vi "main.vi"() -> ()   [LabVIEW 2015]
uses:
  USB Template (LV 8.6)/Car Wash/Controls/Car Wash Indicators.ctl
  USB Template (LV 8.6)/Car Wash/Controls/Wash Options.ctl
  controls/state.ctl
  controls/wash indicators.ctl
  controls/times.ctl
  controls/timer state.ctl
panel:
  out "error out":errorcluster
  in  "error in":errorcluster
  in  "Wash Options":T1
  in  "Start":bool
  out "Elapsed Time":dbl format="%0.2f"
  in  "stop":bool
  out "Wash Entry":bool
  in  "Car Position Slider":u8(slide) max=3 scale=0.0..4.0
  out "Car Wash Indicators":T2
  # "Entry Console"
  # "Car Wash Display"
  # "Car Position Simulation"
  # "Pre-Soak\nH-P Wash\nL-P Wax\nSpot Free Rinse"
  # "Underbody Wash\nBug Remover"
  # "Tire Shine\nAir Dry"
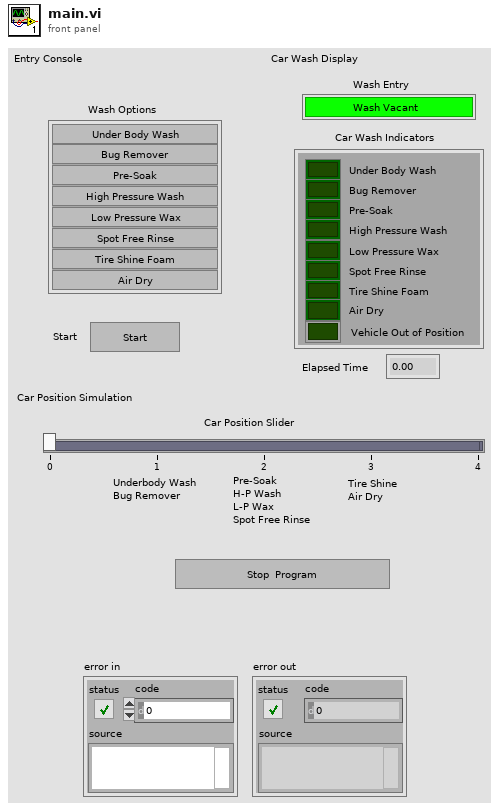
[diagram p1: front panel]
types:
  T1 = typedef "Wash Options.ctl" = cluster{"Underbody Wash":bool, "Bug Remover":bool, "Pre-Soak":bool, "High Pressure Wash":bool, "Low Pressure Wax":bool, "Spot Free Rinse":bool, "Tire Shine Foam":bool, "Air Dry":bool}
  T2 = typedef "Car Wash Indicators.ctl" = cluster{"Under Body Wash":bool, "Bug Remover":bool, "Pre-Soak":bool, "High Pressure Wash":bool, "Low Pressure Wax":bool, "Spot Free Rinse":bool, "Tire Shine Foam":bool, "Air Dry":bool, "Vehicle Out of Position":bool}
  T3 = typedef "state.ctl" = enum16{"Error", "Reset", "Exit", "Next state", "End", "Idle", "UBW", "Bug Remover", "Pre-Soak", "HPW", "LPW", "SFR", "TSF", "Air Dry", "Initialize"}
  T4 = enum8{"Enabled", "Disabled", "Disabled and Grayed Out"}
  T5 = typedef "timer state.ctl" = enum16{"Stop", "Pause", "Start"}
  T6 = typedef "wash indicators.ctl" = cluster{"Car Wash Indicators ":T2, "Wash Entry ":bool, "Elapsed Time ":dbl, "times":T7}
  T7 = typedef "times.ctl" = cluster{"Under Body Wash":dbl, "Bug Remover":dbl, "Pre-Soak":dbl, "High Pressure Wash ":dbl, "Low Pressure Wax":dbl, "Spot Free Rinse":dbl, "Tire Shine Foam":dbl, "Air Dry":dbl}
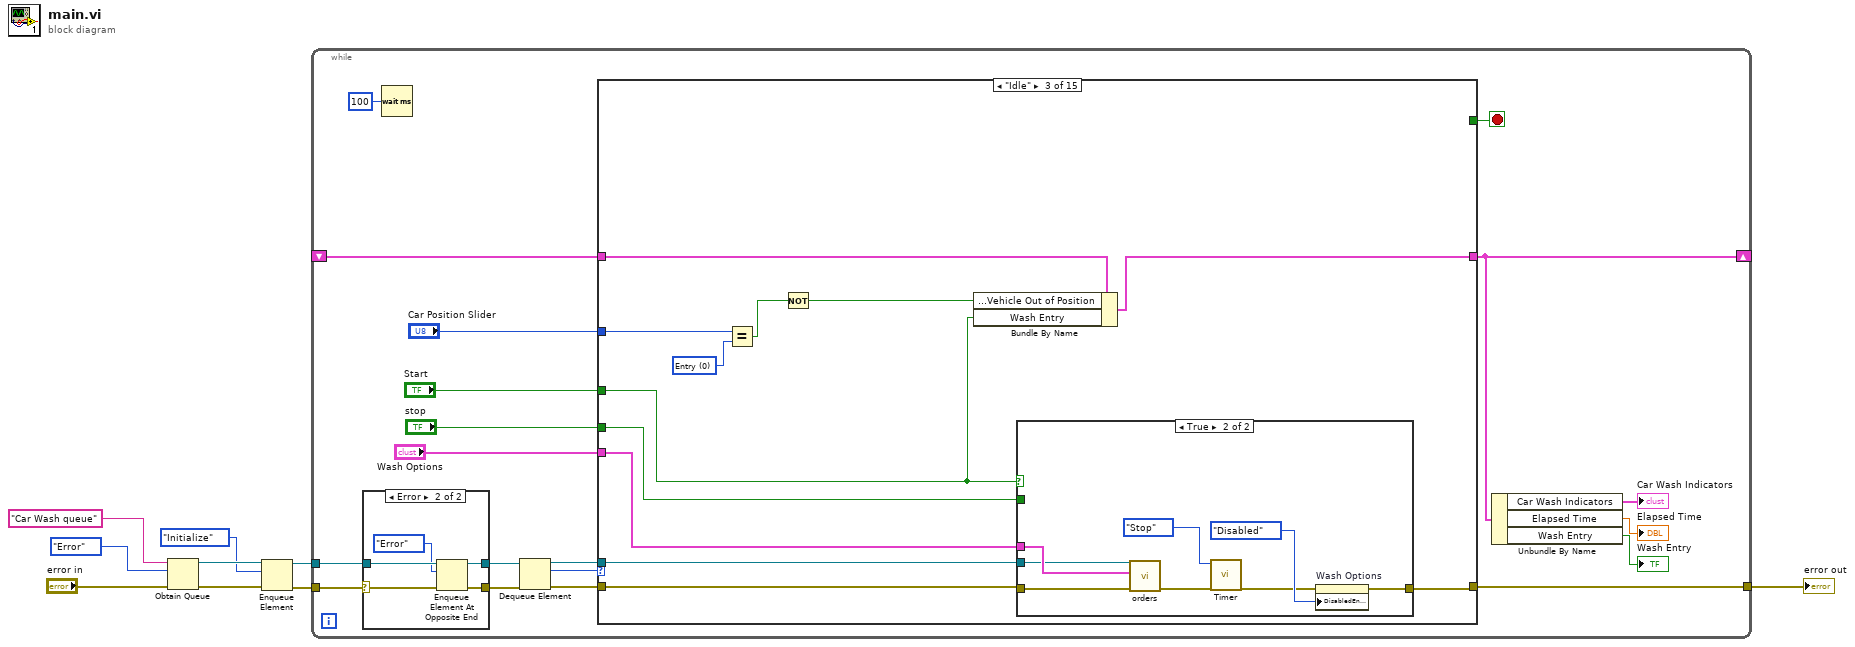
[diagram p0: block diagram]
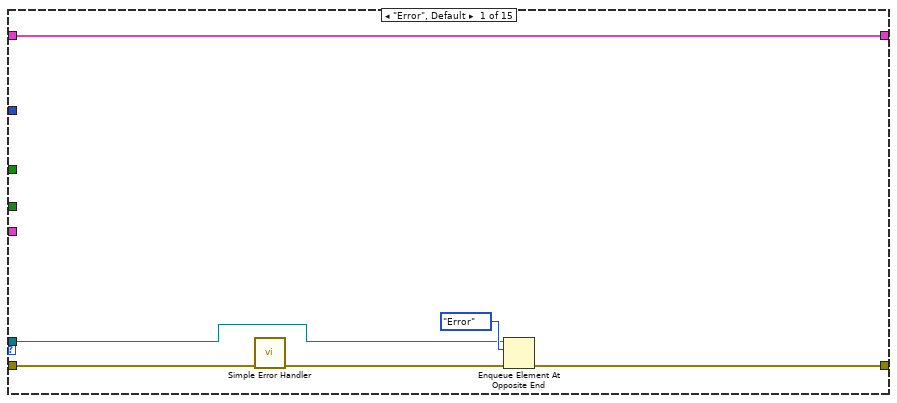
[diagram p3: hidden frame]
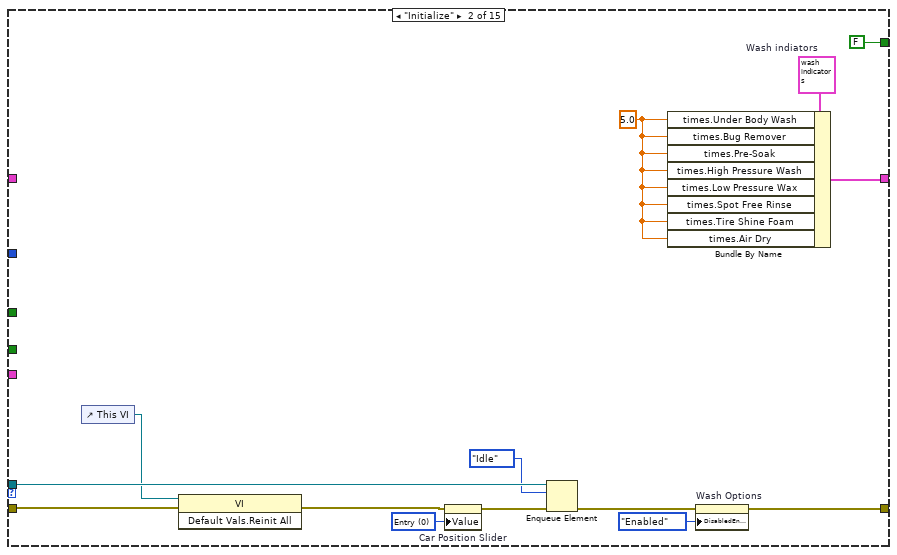
[diagram p4: hidden frame]
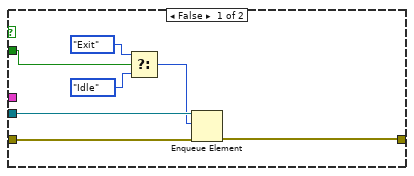
[diagram p5: hidden frame]
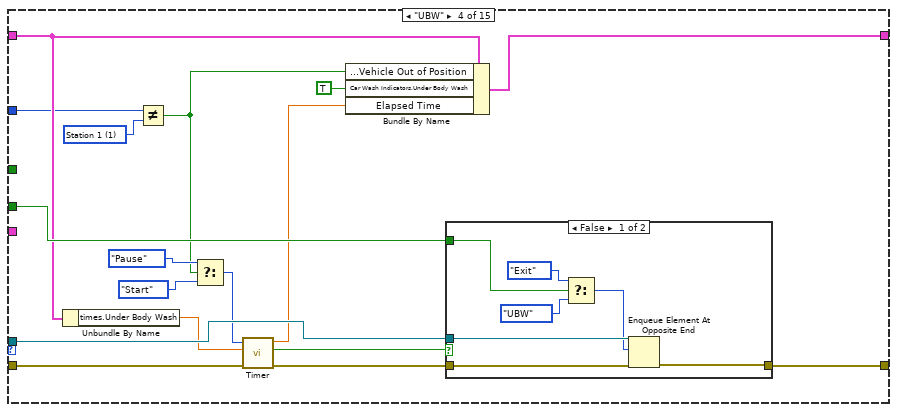
[diagram p6: hidden frame]
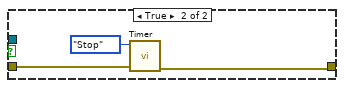
[diagram p7: hidden frame]
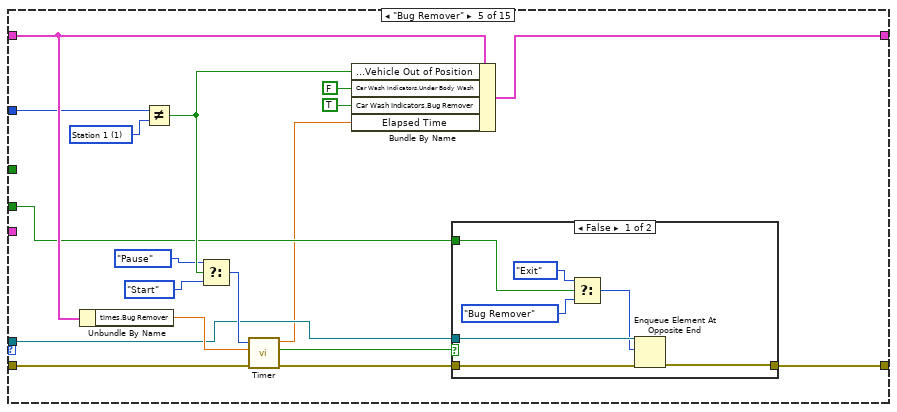
[diagram p8: hidden frame]
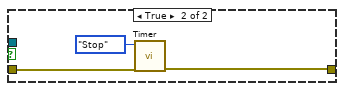
[diagram p9: hidden frame]
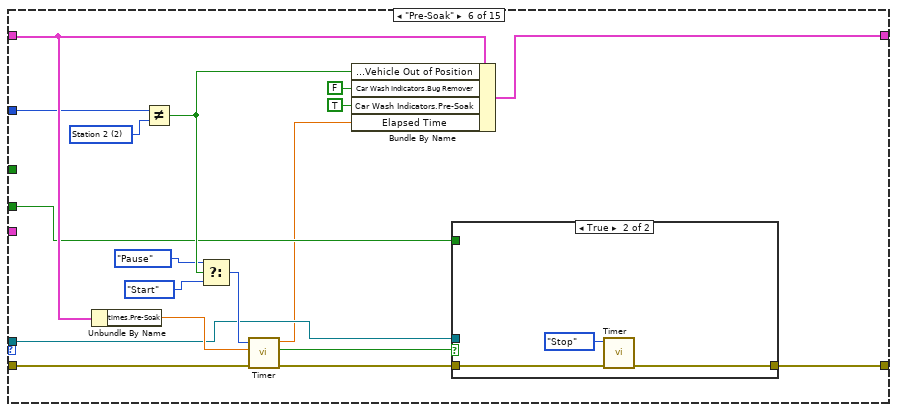
[diagram p10: hidden frame]
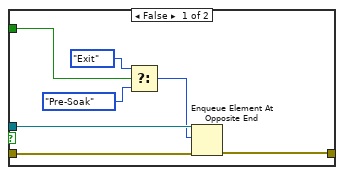
[diagram p11: hidden frame]
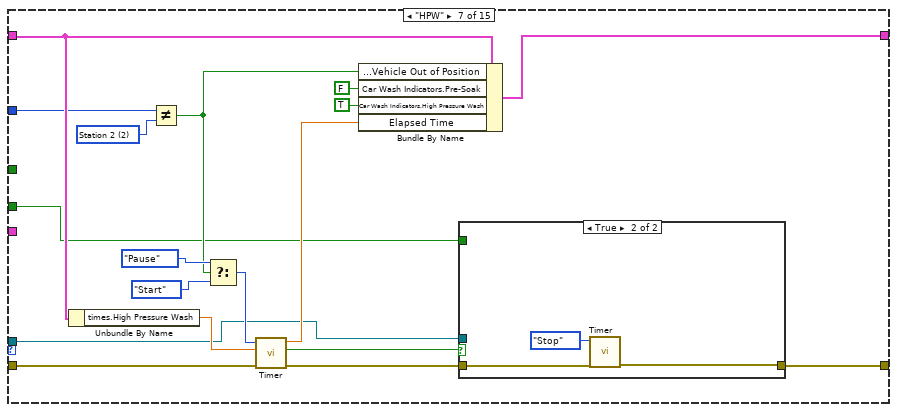
[diagram p12: hidden frame]
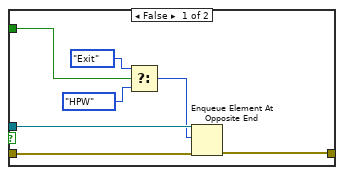
[diagram p13: hidden frame]
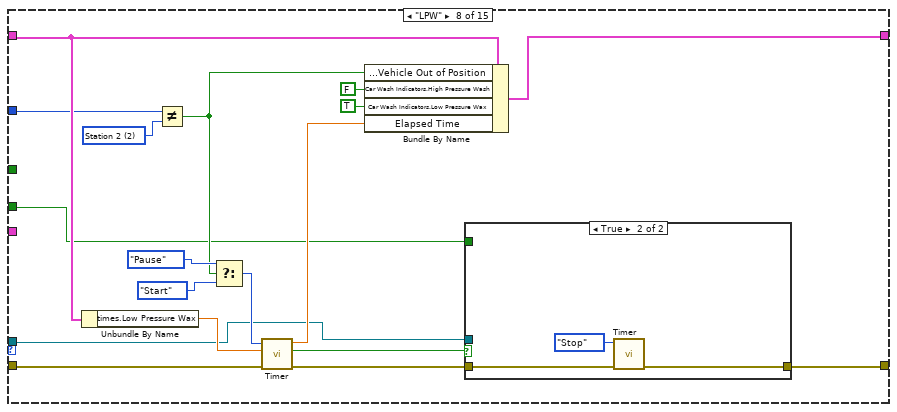
[diagram p14: hidden frame]
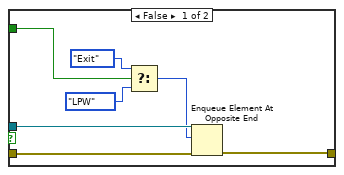
[diagram p15: hidden frame]
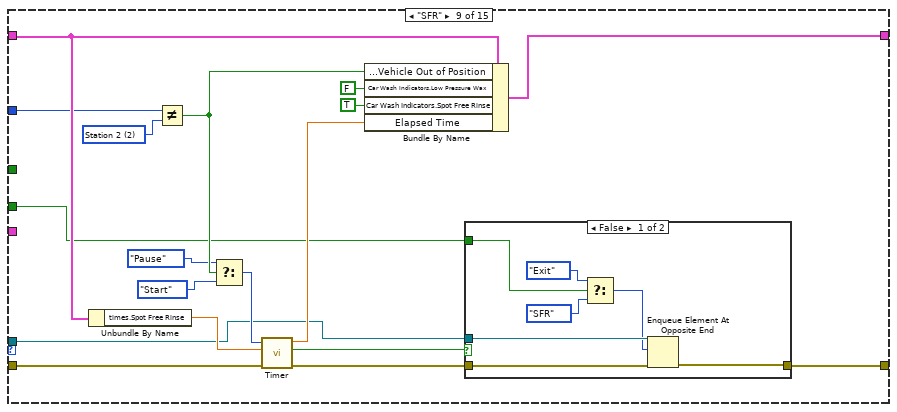
[diagram p16: hidden frame]
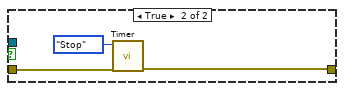
[diagram p17: hidden frame]
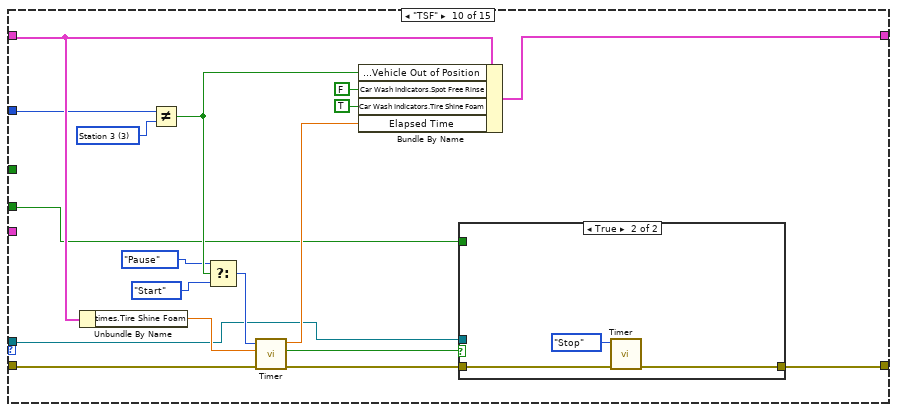
[diagram p18: hidden frame]
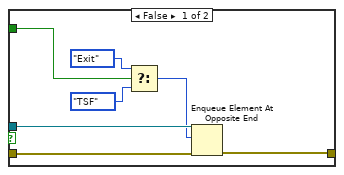
[diagram p19: hidden frame]
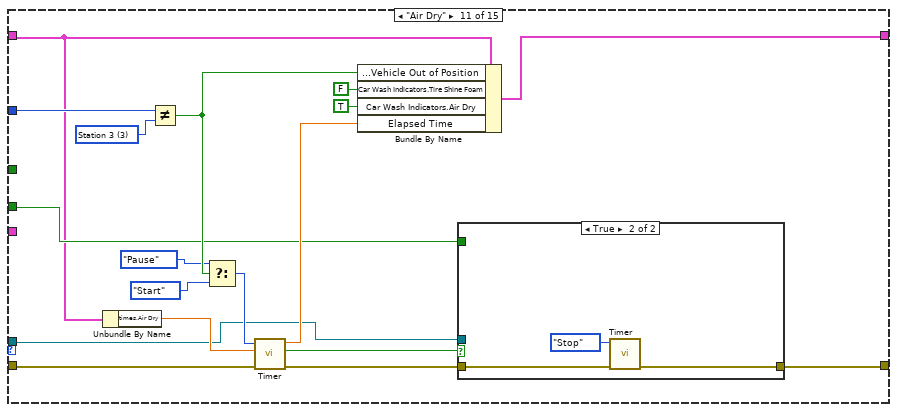
[diagram p20: hidden frame]
diagram:
  n1 = Obtain Queue(name (unnamed)="Car Wash queue", element data type=state."Error" ("state"), error in (no error)="error in") -> (queue out=w3:refnum<queue>, error out=w7:errorcluster)  [unwired: 2 in, 1 out]
  n2 = Enqueue Element(queue=w3, element=state."Initialize" ("state"), error in (no error)=w7) -> (queue out=w1:refnum<queue>, error out=w6:errorcluster)  [unwired: 1 in, 1 out]
  n3 = while {
    tunnel: [w28] -> w9
    tunnel: w6 -> [w18]
    tunnel: w1 -> [w15]
    shift-right: [w14] -> _
    shift-left: _ -> [w21]
    stop <- w24 stop-if-true
    n4 = case shown="Error" w18 {
      selector: w18 -> [w30 w35]
      tunnel: [w30 w34] -> w17
      tunnel: [w29 w33] -> w16
      tunnel: w15 -> [w29 w32]
      frame No Error {
      }
      frame Error {
        n5 = Enqueue Element At Opposite End(queue=w32, element=state."Error" ("state"), error in (no error)=w35) -> (queue out=w33:refnum<queue>, error out=w34:errorcluster)  [unwired: 1 in, 1 out]
      }
    }
    n6 = Wait (ms)(milliseconds to wait=u32 100) -> ()  [unwired: 1 out]
    n7 = Dequeue Element(queue=w16, error in (no error)=w17) -> (queue out=w26:refnum<queue>, element=w25:T3, error out=w27:errorcluster)  [unwired: 1 in, 1 out]
    n8 = case shown="\"Idle\"" w25 {
      tunnel: w27 -> [w41 w44 w66 w97 w117 w143 w171 w198 w227 w255 w284 w308 w313 w319 w347]
      tunnel: [w37 w49 w67 w99 w118 w144 w166 w196 w225 w253 w283 w308 w313 w318 w342] -> w28
      tunnel: w26 -> [w38 w52 w64 w95 w116 w142 w170 w197 w226 w254 w278 _ _ w315 w345]
      tunnel: [_ FALSE _ _ _ _ _ _ _ _ _ TRUE _ _ _] -> w24
      tunnel: [w36 w45 w58 w92 w114 w145 w167 w199 w224 w252 w279 w307 w311 w314 w340] -> w14
      tunnel: "Wash Options" -> [_ _ w65 _ _ _ _ _ _ _ _ _ _ _ _]
      tunnel: "Start" -> [_ _ w56 _ _ _ _ _ _ _ _ _ _ _ _]
      tunnel: w21 -> [w36 _ w61 w91 w115 w146 w172 w200 w228 w256 w280 w307 w312 w316 w340]
      tunnel: "stop" -> [_ _ w62 w98 w112 w141 w169 w195 w223 w251 w282 _ _ _ _]
      tunnel: "Car Position Slider" -> [_ _ w57 w87 w113 w140 w168 w194 w222 w250 w281 _ _ w320 _]
      frame "Error", Default {
        n9 = call <vilib>:"Simple Error Handler.vi"("error in (no error)"=w41) -> ("error out"=w39:errorcluster)  [unwired: 4 in, 4 out]
        n10 = Enqueue Element At Opposite End(queue=w38, element=state."Error" ("state"), error in (no error)=w39) -> (error out=w37:errorcluster)  [unwired: 1 in, 2 out]
      }
      frame "Initialize" {
        w46 = 5.0 ("times.Under Body Wash")
        w54 = u8 0 items=["Entry", "Station 1", "Station 2", "Station 3", "Exit"] ("Car Position Slider")
        w47 = T6 {"Car Wash Indicators "={"Under Body Wash"=FALSE, "Bug Remover"=FALSE, "Pre-Soak"=FALSE, "High Pressure Wash"=FALSE, "Low Pressure Wax"=FALSE, "Spot Free Rinse"=FALSE, "Tire Shine Foam"=FALSE, "Air Dry"=FALSE, "Vehicle Out of Position"=FALSE}, "Wash Entry "=FALSE, "Elapsed Time "=0.0, "times"={"Under Body Wash"=0.0, "Bug Remover"=0.0, "Pre-Soak"=0.0, "High Pressure Wash "=0.0, "Low Pressure Wax"=0.0, "Spot Free Rinse"=0.0, "Tire Shine Foam"=0.0, "Air Dry"=0.0}}  # Wash indiators
        n11 = control-ref of="This VI"() -> (w42:refnum<vi>)
        n12 = invoke class="VI" method="Default Vals.Reinit All"(reference=w42, error in=w44) -> (error out=w43:errorcluster)  [unwired: 1 in, 2 out]
        n13 = property on="Car Position Slider" class="Slide (strict)"(error in=w43, "Value"=w54) -> (error out=w53:errorcluster)  [unwired: 1 in, 1 out]
        n14 = Enqueue Element(queue=w52, element=state."Idle" ("state"), error in (no error)=w53) -> (error out=w50:errorcluster)  [unwired: 1 in, 2 out]
        n15 = Bundle By Name(cluster=w47, "times.Under Body Wash"=w46, "times.Bug Remover"=w46, "times.Pre-Soak"=w46, "times.High Pressure Wash"=w46, "times.Low Pressure Wax"=w46, "times.Spot Free Rinse"=w46, "times.Tire Shine Foam"=w46, "times.Air Dry"=w46) -> (w45:T6)
        n16 = property on="Wash Options" class="Clust (strict)"(error in=w50, "DisabledEnum"=T4."Enabled" ("Disabled")) -> (error out=w49:errorcluster)  [unwired: 1 in, 1 out]
      }
      frame "Idle" {
        w63 = u8 0 items=["Entry", "Station 1", "Station 2", "Station 3", "Exit"] ("Car Position Slider")
        n17 = Equal?(x=w57, y=w63) -> (x = y?=w59:bool)
        n18 = Not(x=w59) -> (.not. x?=w60:bool)
        n19 = Bundle By Name(cluster=w61, "Car Wash Indicators.Vehicle Out of Position"=w60, "Wash Entry"=w56) -> (w58:T6)
        n20 = case shown="True" w56 {
          tunnel: w66 -> [w74 w82]
          tunnel: [w68 w75] -> w67
          tunnel: w65 -> [_ w81]
          tunnel: w64 -> [w73 w80]
          tunnel: w62 -> [w72 _]
          frame False {
            n21 = Select(t=state."Exit" ("state"), s=w72, f=state."Idle" ("state")) -> (s? t:f=w69:T3)
            n22 = Enqueue Element(queue=w73, element=w69, error in (no error)=w74) -> (error out=w68:errorcluster)  [unwired: 1 in, 2 out]
          }
          frame True {
            n23 = call "orders.vi"("error in (no error)"=w82, "Wash Options"=w81, "Queue in"=w80) -> ("error out"=w79:errorcluster)  [unwired: 7 in, 1 out]
            n24 = call "Timer.vi"("error in"=w79, "timer state"=timer_state."Stop") -> ("error out"=w76:errorcluster)  [unwired: 7 in, 2 out]
            n25 = property on="Wash Options" class="Clust (strict)"(error in=w76, "DisabledEnum"=T4."Disabled" ("Disabled")) -> (error out=w75:errorcluster)  [unwired: 1 in, 1 out]
          }
        }
      }
      frame "UBW" {
        w88 = u8 1 items=["Entry", "Station 1", "Station 2", "Station 3", "Exit"] ("Car Position Slider")
        n26 = Unbundle By Name(w91) -> ("times.Under Body Wash"=w90:dbl)
        n27 = Not Equal?(x=w87, y=w88) -> (x != y?=w83:bool)
        n28 = Select(t=timer_state."Pause" ("timer state"), s=w83, f=timer_state."Start" ("timer state")) -> (s? t:f=w84:T5)
        n29 = call "Timer.vi"("error in"=w97, "limit"=w90, "timer state"=w84) -> ("error out"=w96:errorcluster, "limit out"=w94:bool, "elapsed"=w89:dbl)  [unwired: 6 in]
        n30 = Bundle By Name(cluster=w91, "Car Wash Indicators.Vehicle Out of Position"=w83, "Car Wash Indicators.Under Body Wash"=TRUE ("Car Wash Indicators .Under Body Wash"), "Elapsed Time"=w89) -> (w92:T6)
        n31 = case shown="False" w94 {
          tunnel: w96 -> [w106 w108]
          tunnel: [w105 w107] -> w99
          tunnel: w95 -> [w104 _]
          tunnel: w98 -> [w103 _]
          frame False {
            n32 = Select(t=state."Exit" ("state"), s=w103, f=state."UBW" ("state")) -> (s? t:f=w100:T3)
            n33 = Enqueue Element At Opposite End(queue=w104, element=w100, error in (no error)=w106) -> (error out=w105:errorcluster)  [unwired: 1 in, 2 out]
          }
          frame True {
            n34 = call "Timer.vi"("error in"=w108, "timer state"=timer_state."Stop") -> ("error out"=w107:errorcluster)  [unwired: 7 in, 2 out]
          }
        }
      }
      frame "Bug Remover" {
        w123 = u8 1 items=["Entry", "Station 1", "Station 2", "Station 3", "Exit"] ("Car Position Slider")
        n35 = Unbundle By Name(w115) -> ("times.Bug Remover"=w122:dbl)
        n36 = Not Equal?(x=w113, y=w123) -> (x != y?=w127:bool)
        n37 = Select(t=timer_state."Pause" ("timer state"), s=w127, f=timer_state."Start" ("timer state")) -> (s? t:f=w126:T5)
        n38 = call "Timer.vi"("error in"=w117, "limit"=w122, "timer state"=w126) -> ("error out"=w119:errorcluster, "limit out"=w120:bool, "elapsed"=w111:dbl)  [unwired: 6 in]
        n39 = Bundle By Name(cluster=w115, "Car Wash Indicators.Vehicle Out of Position"=w127, "Car Wash Indicators.Under Body Wash"=FALSE ("Car Wash Indicators .Under Body Wash"), "Car Wash Indicators.Bug Remover"=TRUE ("Car Wash Indicators .Bug Remover"), "Elapsed Time"=w111) -> (w114:T6)
        n40 = case shown="False" w120 {
          tunnel: w119 -> [w134 w136]
          tunnel: [w133 w135] -> w118
          tunnel: w116 -> [w132 _]
          tunnel: w112 -> [w131 _]
          frame False {
            n41 = Select(t=state."Exit" ("state"), s=w131, f=state."Bug Remover" ("state")) -> (s? t:f=w128:T3)
            n42 = Enqueue Element At Opposite End(queue=w132, element=w128, error in (no error)=w134) -> (error out=w133:errorcluster)  [unwired: 1 in, 2 out]
          }
          frame True {
            n43 = call "Timer.vi"("error in"=w136, "timer state"=timer_state."Stop") -> ("error out"=w135:errorcluster)  [unwired: 7 in, 2 out]
          }
        }
      }
      frame "Pre-Soak" {
        w151 = u8 2 items=["Entry", "Station 1", "Station 2", "Station 3", "Exit"] ("Car Position Slider")
        n44 = Unbundle By Name(w146) -> ("times.Pre-Soak"=w150:dbl)
        n45 = Not Equal?(x=w140, y=w151) -> (x != y?=w155:bool)
        n46 = Select(t=timer_state."Pause" ("timer state"), s=w155, f=timer_state."Start" ("timer state")) -> (s? t:f=w154:T5)
        n47 = call "Timer.vi"("error in"=w143, "limit"=w150, "timer state"=w154) -> ("error out"=w147:errorcluster, "limit out"=w148:bool, "elapsed"=w139:dbl)  [unwired: 6 in]
        n48 = Bundle By Name(cluster=w146, "Car Wash Indicators.Vehicle Out of Position"=w155, "Car Wash Indicators.Bug Remover"=FALSE ("Car Wash Indicators .Under Body Wash"), "Car Wash Indicators.Pre-Soak"=TRUE ("Car Wash Indicators .Pre-Soak"), "Elapsed Time"=w139) -> (w145:T6)
        n49 = case shown="True" w148 {
          tunnel: w147 -> [w162 w164]
          tunnel: [w161 w163] -> w144
          tunnel: w142 -> [w160 _]
          tunnel: w141 -> [w159 _]
          frame False {
            n50 = Select(t=state."Exit" ("state"), s=w159, f=state."Pre-Soak" ("state")) -> (s? t:f=w156:T3)
            n51 = Enqueue Element At Opposite End(queue=w160, element=w156, error in (no error)=w162) -> (error out=w161:errorcluster)  [unwired: 1 in, 2 out]
          }
          frame True {
            n52 = call "Timer.vi"("error in"=w164, "timer state"=timer_state."Stop") -> ("error out"=w163:errorcluster)  [unwired: 7 in, 2 out]
          }
        }
      }
      frame "HPW" {
        w177 = u8 2 items=["Entry", "Station 1", "Station 2", "Station 3", "Exit"] ("Car Position Slider")
        n53 = Unbundle By Name(w172) -> ("times.High Pressure Wash"=w178:dbl)
        n54 = Not Equal?(x=w168, y=w177) -> (x != y?=w173:bool)
        n55 = Select(t=timer_state."Pause" ("timer state"), s=w173, f=timer_state."Start" ("timer state")) -> (s? t:f=w174:T5)
        n56 = call "Timer.vi"("error in"=w171, "limit"=w178, "timer state"=w174) -> ("error out"=w181:errorcluster, "limit out"=w180:bool, "elapsed"=w182:dbl)  [unwired: 6 in]
        n57 = Bundle By Name(cluster=w172, "Car Wash Indicators.Vehicle Out of Position"=w173, "Car Wash Indicators.Pre-Soak"=FALSE ("Car Wash Indicators .Under Body Wash"), "Car Wash Indicators.High Pressure Wash"=TRUE ("Car Wash Indicators .Pre-Soak"), "Elapsed Time"=w182) -> (w167:T6)
        n58 = case shown="True" w180 {
          tunnel: w181 -> [w190 w192]
          tunnel: [w189 w191] -> w166
          tunnel: w170 -> [w188 _]
          tunnel: w169 -> [w187 _]
          frame False {
            n59 = Select(t=state."Exit" ("state"), s=w187, f=state."HPW" ("state")) -> (s? t:f=w184:T3)
            n60 = Enqueue Element At Opposite End(queue=w188, element=w184, error in (no error)=w190) -> (error out=w189:errorcluster)  [unwired: 1 in, 2 out]
          }
          frame True {
            n61 = call "Timer.vi"("error in"=w192, "timer state"=timer_state."Stop") -> ("error out"=w191:errorcluster)  [unwired: 7 in, 2 out]
          }
        }
      }
      frame "LPW" {
        w205 = u8 2 items=["Entry", "Station 1", "Station 2", "Station 3", "Exit"] ("Car Position Slider")
        n62 = Unbundle By Name(w200) -> ("times.Low Pressure Wax"=w206:dbl)
        n63 = Not Equal?(x=w194, y=w205) -> (x != y?=w201:bool)
        n64 = Select(t=timer_state."Pause" ("timer state"), s=w201, f=timer_state."Start" ("timer state")) -> (s? t:f=w202:T5)
        n65 = call "Timer.vi"("error in"=w198, "limit"=w206, "timer state"=w202) -> ("error out"=w209:errorcluster, "limit out"=w208:bool, "elapsed"=w210:dbl)  [unwired: 6 in]
        n66 = Bundle By Name(cluster=w200, "Car Wash Indicators.Vehicle Out of Position"=w201, "Car Wash Indicators.High Pressure Wash"=FALSE ("Car Wash Indicators .Under Body Wash"), "Car Wash Indicators.Low Pressure Wax"=TRUE ("Car Wash Indicators .Pre-Soak"), "Elapsed Time"=w210) -> (w199:T6)
        n67 = case shown="True" w208 {
          tunnel: w209 -> [w218 w220]
          tunnel: [w217 w219] -> w196
          tunnel: w197 -> [w216 _]
          tunnel: w195 -> [w215 _]
          frame False {
            n68 = Select(t=state."Exit" ("state"), s=w215, f=state."LPW" ("state")) -> (s? t:f=w212:T3)
            n69 = Enqueue Element At Opposite End(queue=w216, element=w212, error in (no error)=w218) -> (error out=w217:errorcluster)  [unwired: 1 in, 2 out]
          }
          frame True {
            n70 = call "Timer.vi"("error in"=w220, "timer state"=timer_state."Stop") -> ("error out"=w219:errorcluster)  [unwired: 7 in, 2 out]
          }
        }
      }
      frame "SFR" {
        w235 = u8 2 items=["Entry", "Station 1", "Station 2", "Station 3", "Exit"] ("Car Position Slider")
        n71 = Unbundle By Name(w228) -> ("times.Spot Free Rinse"=w234:dbl)
        n72 = Not Equal?(x=w222, y=w235) -> (x != y?=w239:bool)
        n73 = Select(t=timer_state."Pause" ("timer state"), s=w239, f=timer_state."Start" ("timer state")) -> (s? t:f=w238:T5)
        n74 = call "Timer.vi"("error in"=w227, "limit"=w234, "timer state"=w238) -> ("error out"=w231:errorcluster, "limit out"=w232:bool, "elapsed"=w230:dbl)  [unwired: 6 in]
        n75 = Bundle By Name(cluster=w228, "Car Wash Indicators.Vehicle Out of Position"=w239, "Car Wash Indicators.Low Pressure Wax"=FALSE ("Car Wash Indicators .Under Body Wash"), "Car Wash Indicators.Spot Free Rinse"=TRUE ("Car Wash Indicators .Pre-Soak"), "Elapsed Time"=w230) -> (w224:T6)
        n76 = case shown="False" w232 {
          tunnel: w231 -> [w246 w249]
          tunnel: [w245 w248] -> w225
          tunnel: w226 -> [w244 _]
          tunnel: w223 -> [w243 _]
          frame False {
            n77 = Select(t=state."Exit" ("state"), s=w243, f=state."SFR" ("state")) -> (s? t:f=w240:T3)
            n78 = Enqueue Element At Opposite End(queue=w244, element=w240, error in (no error)=w246) -> (error out=w245:errorcluster)  [unwired: 1 in, 2 out]
          }
          frame True {
            n79 = call "Timer.vi"("error in"=w249, "timer state"=timer_state."Stop") -> ("error out"=w248:errorcluster)  [unwired: 7 in, 2 out]
          }
        }
      }
      frame "TSF" {
        w263 = u8 3 items=["Entry", "Station 1", "Station 2", "Station 3", "Exit"] ("Car Position Slider")
        n80 = Unbundle By Name(w256) -> ("times.Tire Shine Foam"=w262:dbl)
        n81 = Not Equal?(x=w250, y=w263) -> (x != y?=w267:bool)
        n82 = Select(t=timer_state."Pause" ("timer state"), s=w267, f=timer_state."Start" ("timer state")) -> (s? t:f=w266:T5)
        n83 = call "Timer.vi"("error in"=w255, "limit"=w262, "timer state"=w266) -> ("error out"=w259:errorcluster, "limit out"=w260:bool, "elapsed"=w258:dbl)  [unwired: 6 in]
        n84 = Bundle By Name(cluster=w256, "Car Wash Indicators.Vehicle Out of Position"=w267, "Car Wash Indicators.Spot Free Rinse"=FALSE ("Car Wash Indicators .Under Body Wash"), "Car Wash Indicators.Tire Shine Foam"=TRUE ("Car Wash Indicators .Pre-Soak"), "Elapsed Time"=w258) -> (w252:T6)
        n85 = case shown="True" w260 {
          tunnel: w259 -> [w274 w276]
          tunnel: [w273 w275] -> w253
          tunnel: w254 -> [w272 _]
          tunnel: w251 -> [w271 _]
          frame False {
            n86 = Select(t=state."Exit" ("state"), s=w271, f=state."TSF" ("state")) -> (s? t:f=w268:T3)
            n87 = Enqueue Element At Opposite End(queue=w272, element=w268, error in (no error)=w274) -> (error out=w273:errorcluster)  [unwired: 1 in, 2 out]
          }
          frame True {
            n88 = call "Timer.vi"("error in"=w276, "timer state"=timer_state."Stop") -> ("error out"=w275:errorcluster)  [unwired: 7 in, 2 out]
          }
        }
      }
      frame "Air Dry" {
        w291 = u8 3 items=["Entry", "Station 1", "Station 2", "Station 3", "Exit"] ("Car Position Slider")
        n89 = Unbundle By Name(w280) -> ("times.Air Dry"=w290:dbl)
        n90 = Not Equal?(x=w281, y=w291) -> (x != y?=w295:bool)
        n91 = Select(t=timer_state."Pause" ("timer state"), s=w295, f=timer_state."Start" ("timer state")) -> (s? t:f=w294:T5)
        n92 = call "Timer.vi"("error in"=w284, "limit"=w290, "timer state"=w294) -> ("error out"=w287:errorcluster, "limit out"=w288:bool, "elapsed"=w286:dbl)  [unwired: 6 in]
        n93 = Bundle By Name(cluster=w280, "Car Wash Indicators.Vehicle Out of Position"=w295, "Car Wash Indicators.Tire Shine Foam"=FALSE ("Car Wash Indicators .Under Body Wash"), "Car Wash Indicators.Air Dry"=TRUE ("Car Wash Indicators .Pre-Soak"), "Elapsed Time"=w286) -> (w279:T6)
        n94 = case shown="True" w288 {
          tunnel: w287 -> [w302 w304]
          tunnel: [w301 w303] -> w283
          tunnel: w278 -> [w300 _]
          tunnel: w282 -> [w299 _]
          frame False {
            n95 = Select(t=state."Exit" ("state"), s=w299, f=state."Air Dry" ("state")) -> (s? t:f=w296:T3)
            n96 = Enqueue Element At Opposite End(queue=w300, element=w296, error in (no error)=w302) -> (error out=w301:errorcluster)  [unwired: 1 in, 2 out]
          }
          frame True {
            n97 = call "Timer.vi"("error in"=w304, "timer state"=timer_state."Stop") -> ("error out"=w303:errorcluster)  [unwired: 7 in, 2 out]
          }
        }
      }
      frame "Exit" {
      }
      frame "Next state" {
        n98 = Bundle By Name(cluster=w312, "Car Wash Indicators"=T2 {"Under Body Wash"=FALSE, "Bug Remover"=FALSE, "Pre-Soak"=FALSE, "High Pressure Wash"=FALSE, "Low Pressure Wax"=FALSE, "Spot Free Rinse"=FALSE, "Tire Shine Foam"=FALSE, "Air Dry"=FALSE, "Vehicle Out of Position"=FALSE}, "Elapsed Time"=0.0) -> (w311:T6)
      }
      frame "End" {
        w321 = u8 4 items=["Entry", "Station 1", "Station 2", "Station 3", "Exit"] ("Car Position Slider")
        n99 = Equal?(x=w320, y=w321) -> (x = y?=w317:bool)
        n100 = case shown="True" w317 {
          tunnel: w319 -> [w326 w331]
          tunnel: [w325 w330] -> w318
          tunnel: w316 -> [w329 w339]
          tunnel: w315 -> [w324 w333]
          tunnel: [w322 w338] -> w314
          frame False {
            n101 = Bundle By Name(cluster=w329, "Car Wash Indicators.Air Dry"=FALSE ("Car Wash Indicators .Air Dry"), "Car Wash Indicators.Vehicle Out of Position"=TRUE ("Car Wash Indicators .Vehicle Out of Position")) -> (w322:T6)
            n102 = Enqueue Element At Opposite End(queue=w324, element=state."End", error in (no error)=w326) -> (error out=w325:errorcluster)  [unwired: 1 in, 2 out]
          }
          frame True {
            n103 = Bundle By Name(cluster=w339, "Car Wash Indicators.Air Dry"=FALSE ("Car Wash Indicators .Air Dry"), "Car Wash Indicators.Vehicle Out of Position"=FALSE ("Car Wash Indicators .Vehicle Out of Position"), "Wash Entry"=FALSE, "Elapsed Time"=0.0) -> (w338:T6)
            n104 = Enqueue Element(queue=w333, element=state."Reset" ("state"), error in (no error)=w331) -> (error out=w330:errorcluster)  [unwired: 1 in, 2 out]
          }
        }
      }
      frame "Reset" {
        w350 = u8 0 items=["Entry", "Station 1", "Station 2", "Station 3", "Exit"] ("Car Position Slider")
        n105 = Enqueue Element At Opposite End(queue=w345, element=state."Idle" ("state"), error in (no error)=w347) -> (error out=w346:errorcluster)  [unwired: 1 in, 2 out]
        n106 = property on="Car Position Slider" class="Slide (strict)"(error in=w346, "Val(Sgnl)"=w350) -> (error out=w349:errorcluster)  [unwired: 1 in, 1 out]
        n107 = property on="Wash Options" class="Clust (strict)"(error in=w349, "DisabledEnum"=T4."Enabled" ("Disabled")) -> (error out=w343:errorcluster)  [unwired: 1 in, 1 out]
        n108 = control-ref of="This VI"() -> (w341:refnum<vi>)
        n109 = invoke class="VI" method="Default Vals.Reinit All"(reference=w341, error in=w343) -> (error out=w342:errorcluster)  [unwired: 1 in, 2 out]
      }
    }
    n110 = Unbundle By Name(w14) -> ("Car Wash Indicators"=→"Car Wash Indicators":T2, "Elapsed Time"=→"Elapsed Time":dbl, "Wash Entry"=→"Wash Entry":bool)
  }
  "error out" <- w9
